vi "Load Config.vi"(8 "error in (no error)":errorcluster, 9 "Default Value in":variant, 10 "Section":string, 11 "Project in":refnum<class "Project.lvclass">) -> (0 "error out":errorcluster, 1 "Value out":variant, 3 "Project out":refnum<class "Project.lvclass">)   [LabVIEW 2015, in "Project.lvclass"]
uses:
  Project.lvclass
  <vilib>/Utility/config.llb/NI_LVConfig.lvlib
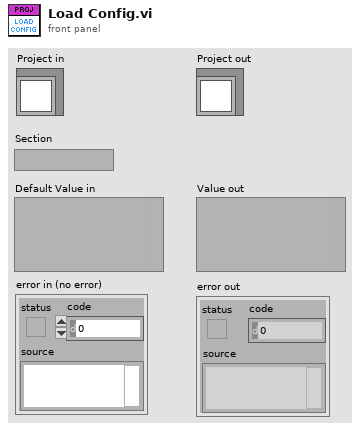
[diagram p1: front panel]
types:
  T1 = typedef "NI_LVConfig.lvlib/Config Data RefNum.ctl" = refnum<k1>
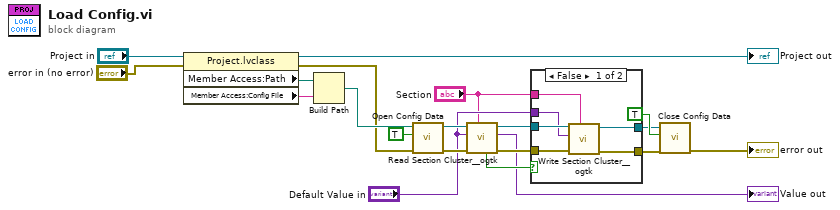
[diagram p0: block diagram]
diagram:
  n1 = property class="Project.lvclass"(reference="Project in", error in="error in (no error)") -> (reference out=→"Project out":refnum<class "Project.lvclass">, error out=w7:errorcluster, "Member Access:Path"=w10:path, "Member Access:Config File"=w9:string)
  n2 = Build Path(base path=w10, name or relative path=w9) -> (appended path=w8:path)
  n3 = call <vilib>:"Open Config Data.vi"("error in (no error)"=w7, "create file if necessary (T)"=TRUE, "configuration file path"=w8) -> ("error out"=w19:errorcluster, "refnum"=w18:T1)  [unwired: 6 in, 1 out]
  n4 = call <userlib>:"Read Section Cluster__ogtk.vi"("section (optional)"="Section", "error in (no error)"=w19, "Section Formatted Cluster Type"="Default Value in", "refnum"=w18) -> ("error out"=w14:errorcluster, "Section Formatted Cluster"=→"Value out":variant, "dup refnum"=w15:T1, "any found?"=w16:bool)  [unwired: 3 in, 1 out]
  n5 = case shown="False" w16 {
    tunnel: w15 -> [w26 w28]
    tunnel: w14 -> [w25 w27]
    tunnel: "Section" -> [w24 _]
    tunnel: "Default Value in" -> [w23 _]
    tunnel: [w22 w28] -> w13
    tunnel: [w21 w27] -> w12
    frame False {
      n6 = call <userlib>:"Write Section Cluster__ogtk.vi"("section (optional)"=w24, "error in (no error)"=w25, "Section Formatted Cluster"=w23, "refnum"=w26) -> ("error out"=w21:errorcluster, "dup refnum"=w22:T1)  [unwired: 6 in]
    }
    frame True {
    }
  }
  n7 = call <vilib>:"Close Config Data.vi"("error in (no error)"=w12, "write file if changed (T)"=TRUE, "refnum"=w13) -> ("error out"=→"error out":errorcluster)  [unwired: 7 in, 1 out]
